vi "Float32Array Create.vi"(8 "error in (no error)":errorcluster, 11 "SGL array in":sgl[](array[numeric])) -> (0 "error out":errorcluster, 3 "Float32Array DVR out":refnum<data-value>)   [LabVIEW 2012, in "MDSplus.lvlib"]
uses:
  <vilib>/MDSplus/Library/MDSplus.lvlib
  <vilib>/MDSplus/Classes/Data_Class/Array_Class/Float32Array_Class/Float32Array.lvclass
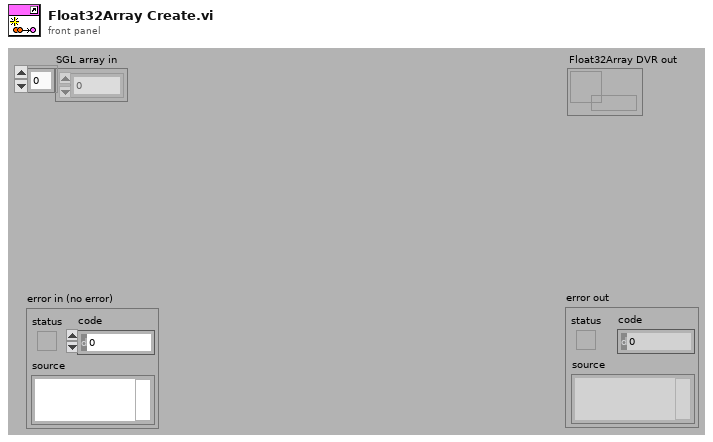
[diagram p1: front panel]
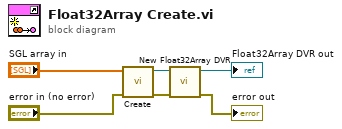
[diagram p0: block diagram]
diagram:
  n1 = call <vilib>:"Create.vi"("error in (no error)"="error in (no error)", "SGL array in"="SGL array in") -> ("error out"=w3:errorcluster, "Float32Array out"=w4:refnum<class "Float32Array.lvclass">)  [unwired: 8 in]
  n2 = call <vilib>:"New Float32Array DVR.vi"("error in (no error)"=w3, "Float32Array in"=w4) -> ("error out"=→"error out":errorcluster, "Float32Array DVR out"=→"Float32Array DVR out":refnum<data-value>)  [unwired: 8 in]
